vi "StopRequest.vi"(8 "ErrorArray In":errorcluster[](array[cluster]), 11 "BusIndex":i8=-1) -> (0 "ErrorArray Out":errorcluster[](array[cluster]))   [LabVIEW 2014, in "TestFramework.lvlib"]
uses:
  TestFramework.lvlib
  Protected/clUserEventType.ctl
  <vilib>/Utility/error.llb/Error Cluster From Error Code.vi
  <vilib>/ErrorRing/Error Ring.xnode
  <userlib>/NIST/NISTErrorLib/NISTErrorLib.lvlib
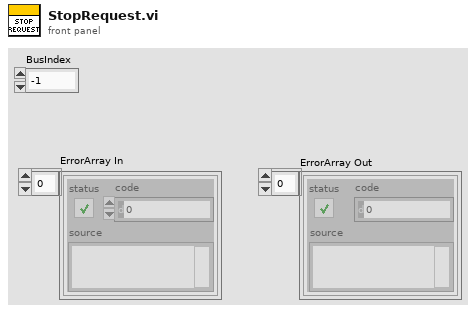
[diagram p1: front panel]
types:
  T1 = typedef "TestFramework.lvlib/clUserEventType.ctl" = cluster{"BusIndex":i8, "Data":variant}
  T2 = typedef "TestFramework.lvlib/clRequestEvents.ctl" = cluster{"StopRequest":refnum<user-event>}
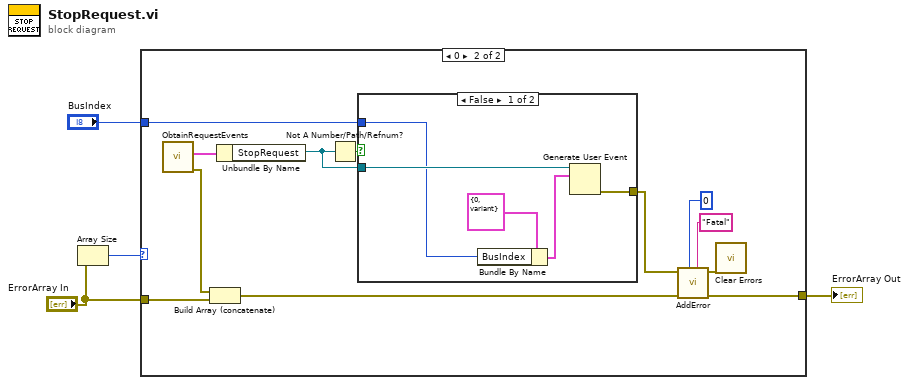
[diagram p0: block diagram]
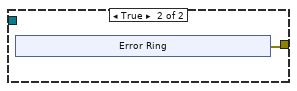
[diagram p3: hidden frame]
diagram:
  n1 = Array Size(array="ErrorArray In") -> (size(s)=w4:i32)
  n2 = case shown="0" w4 {
    tunnel: "BusIndex" -> [_ w14]
    tunnel: "ErrorArray In" -> [w5 w12]
    tunnel: [w5 w6] -> w1
    frame 1, Default {
    }
    frame 0 {
      n3 = call "ObtainRequestEvents.vi"() -> ("ErrorArray Out"=w13:errorcluster[], "clRequestEvents"=w17:T2)  [unwired: 10 in]
      n4 = Build Array (concatenate)(w13, w12) -> (w8:errorcluster[])
      n5 = Unbundle By Name(w17) -> ("StopRequest"=w15:refnum<user-event>)
      n6 = Not A Number/Path/Refnum?(number/path/refnum=w15) -> (NaN/Path/Refnum?=w16:bool)
      n7 = case shown="False" w16 {
        tunnel: w14 -> [w20 _]
        tunnel: w15 -> [w22 _]
        tunnel: [w18 w23] -> w7
        frame False {
          n8 = Bundle By Name(cluster=T1 {"BusIndex"=0, "Data"=variant} ("clEventType"), "BusIndex"=w20) -> (w19:T1)
          n9 = Generate User Event(user event=w22, event data cluster=w19) -> (error out=w18:errorcluster)  [unwired: 2 in, 1 out]
        }
        frame True {
          n10 = xnode "Error Ring"() -> ("error out"=w23:errorcluster)
        }
      }
      n11 = call <userlib>:"AddError.vi"("Severity"="Fatal" ("String"), "Priority"=u8 0, "ErrorArray"=w8, "error in (no error)"=w7) -> ("ErrorArray"=w6:errorcluster[], "error out"=w11:errorcluster)  [unwired: 6 in]
      n12 = call <vilib>:"Clear Errors.vi"("error in (no error)"=w11) -> ()  [unwired: 5 in, 2 out]
    }
  }
  "ErrorArray Out" <- w1
